vi "GLB_PAmonts.vi"() -> ()   [LabVIEW 2014]
panel:
  in  "PAmonts":cluster{"P1":dbl, "P2":dbl, "P3":dbl, "P4":dbl}
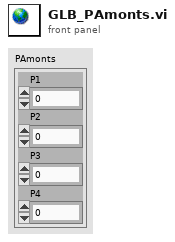
[diagram p1: front panel]
diagram:
